vi "Step Core.vi"(8 "error in (no error)":errorcluster, 11 "Servo MSMT in":refnum<class "Servo MSMT.lvclass">) -> (0 "error out":errorcluster, 3 "Servo MSMT out":refnum<class "Servo MSMT.lvclass">)   [LabVIEW 2018, in "Servo MSMT.lvlib" / "Servo MSMT.lvclass"]
uses:
  Servo MSMT.lvclass
  Plugins/Measurement Interface.lvlibp/Measurement Interface.lvclass
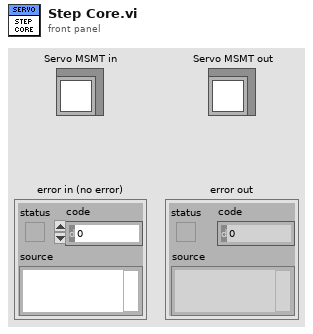
[diagram p1: front panel]
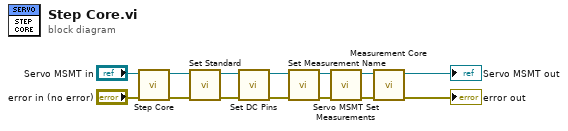
[diagram p0: block diagram]
diagram:
  n1 = call-parent "Step Core.vi"("error in (no error)"="error in (no error)", "Measurement Interface in"="Servo MSMT in") -> ("error out"=w14:errorcluster, "Measurement Interface out"=w8:refnum<class "Servo MSMT.lvclass">)  [unwired: 8 in]
  n2 = call "Set Standard.vi"("error in (no error)"=w14, "Servo MSMT in"=w8) -> ("error out"=w9:errorcluster, "Servo MSMT out"=w3:refnum<class "Servo MSMT.lvclass">)  [unwired: 8 in]
  n3 = call "Set DC Pins.vi"("error in (no error)"=w9, "Servo MSMT in"=w3) -> ("error out"=w4:errorcluster, "Servo MSMT out"=w2:refnum<class "Servo MSMT.lvclass">)  [unwired: 8 in]
  n4 = call-dynamic "Set Measurement Name.vi"("error in (no error)"=w4, "Servo MSMT in"=w2) -> ("error out"=w7:errorcluster, "Servo MSMT out"=w1:refnum<class "Servo MSMT.lvclass">)  [unwired: 8 in]
  n5 = call "Servo MSMT Set Measurements.vi"("error in (no error)"=w7, "Servo MSMT in"=w1) -> ("error out"=w6:errorcluster, "Servo MSMT out"=w5:refnum<class "Servo MSMT.lvclass">)  [unwired: 8 in]
  n6 = call "Measurement Core.vi"("error in (no error)"=w6, "Servo MSMT in"=w5) -> ("error out"=→"error out":errorcluster, "Servo MSMT out"=→"Servo MSMT out":refnum<class "Servo MSMT.lvclass">)  [unwired: 8 in]
